vi "Get Alarm Status.vi"(8 "error in (no error)":errorcluster, 9 "Sample Rate Hz":dbl, 10 "Acquisition Metrics in":T1={"Total_Samples"=0, "RPM"=1000.0}, 11 "data":waveform(dbl)[](array[waveform])) -> (0 "error out":errorcluster, 3 "Alarms":T2)   [LabVIEW 2026, in "Acquisition.lvlib"]
uses:
  Acquisition.lvlib
  Controls/Alarms.ctl
  Controls/Frequency Type.ctl
  Controls/Acquisition Metrics.ctl
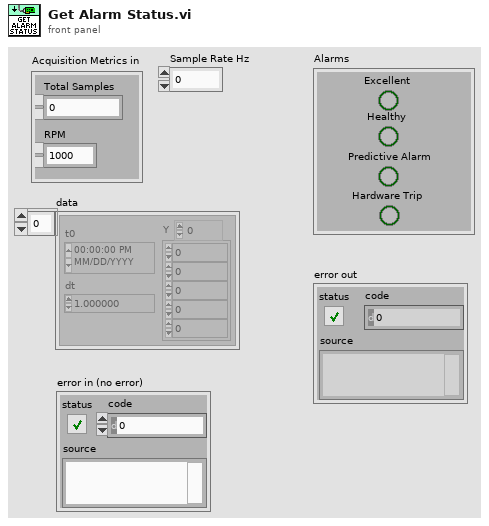
[diagram p1: front panel]
types:
  T1 = typedef "Acquisition.lvlib/Acquisition Metrics.ctl" = cluster{"Total_Samples":i64, "RPM":dbl}
  T2 = typedef "Acquisition.lvlib/Alarms.ctl" = cluster{"Excellent":bool, "Healthy":bool, "Predictive Alarm":bool, "Hardware Trip":bool}
  T3 = typedef "Acquisition.lvlib/Frequency Type.ctl" = enum16{"Calc F_1X", "Calc F_cutoff"}
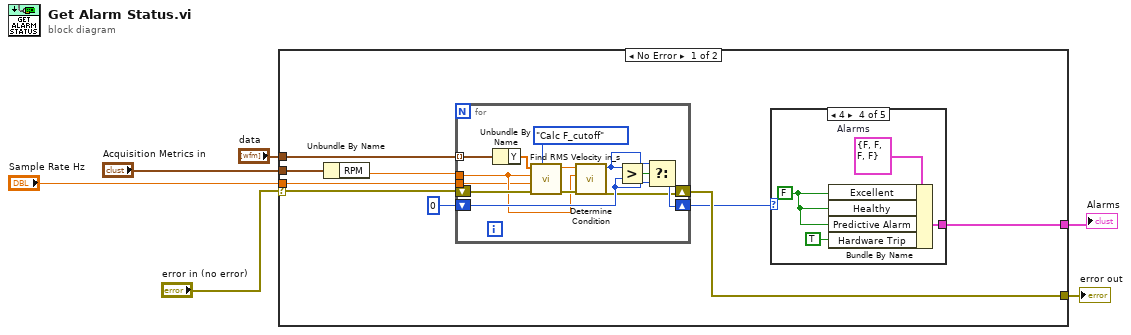
[diagram p0: block diagram]
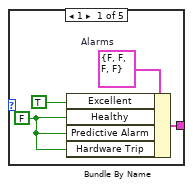
[diagram p2: hidden frame]
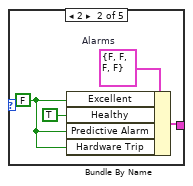
[diagram p3: hidden frame]
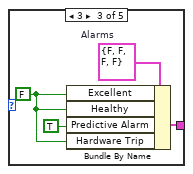
[diagram p4: hidden frame]
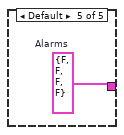
[diagram p5: hidden frame]
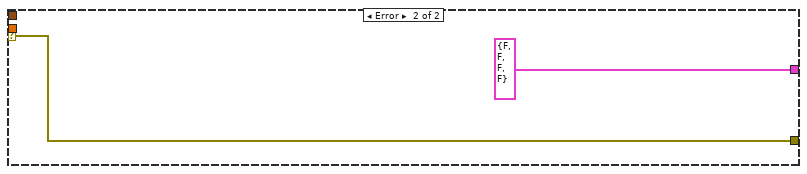
[diagram p6: hidden frame]
diagram:
  n1 = case shown="No Error" "error in (no error)" {
    selector: "error in (no error)" -> [w10 w46]
    tunnel: [w15 w46] -> w6
    tunnel: "data" -> [w14 _]
    tunnel: [w11 T2 {"Excellent"=FALSE, "Healthy"=FALSE, "Predictive Alarm"=FALSE, "Hardware Trip"=FALSE} ("Alarms")] -> w4
    tunnel: "Sample Rate Hz" -> [w9 _]
    tunnel: "Acquisition Metrics in" -> [w8 _]
    frame No Error {
      n2 = Unbundle By Name(w8) -> ("RPM"=w7:dbl)
      n3 = for {
        shift-right: [w24] -> w13
        shift-left: 0 ("Condition") -> [w23]
        tunnel: w14 -> [w21] mode=indexing
        shift-right: [w19] -> w15
        shift-left: w10 -> [w20]
        tunnel: w7 -> [w17]
        tunnel: w9 -> [w16]
        n4 = Unbundle By Name(w21) -> ("Y"=w28:dbl[])
        n5 = call "Find RMS Velocity in_s .vi"("Freq. Type"=Frequency_Type."Calc F_cutoff", "error in (no error)"=w20, "Sample Rate Hz"=w16, "RPM"=w17, "Y"=w28) -> ("error out"=w27:errorcluster, "rms value"=w22:dbl)  [unwired: 5 in]
        n6 = call "Determine Condition.vi"("error in (no error)"=w27, "RPM"=w17, "RMS"=w22) -> ("error out"=w19:errorcluster, "Condition"=w25:i32)  [unwired: 7 in]
        n7 = Greater?(x=w25, y=w23) -> (0:w26:bool)
        n8 = Select(t=w25, s=w26, f=w23) -> (s? t:f=w24:i32)
      }
      n9 = case shown="4" w13 {
        tunnel: [w31 w35 w39 w43 w45] -> w11
        frame 1 {
          w30 = FALSE ("Excellent")
          w32 = T2 {"Excellent"=FALSE, "Healthy"=FALSE, "Predictive Alarm"=FALSE, "Hardware Trip"=FALSE}  # Alarms
          n10 = Bundle By Name(cluster=w32, "Excellent"=TRUE ("Healthy"), "Healthy"=w30, "Predictive Alarm"=w30, "Hardware Trip"=w30) -> (w31:T2)
        }
        frame 2 {
          w34 = FALSE ("Excellent")
          w36 = T2 {"Excellent"=FALSE, "Healthy"=FALSE, "Predictive Alarm"=FALSE, "Hardware Trip"=FALSE}  # Alarms
          n11 = Bundle By Name(cluster=w36, "Excellent"=w34, "Healthy"=TRUE, "Predictive Alarm"=w34, "Hardware Trip"=w34) -> (w35:T2)
        }
        frame 3 {
          w38 = FALSE ("Excellent")
          w40 = T2 {"Excellent"=FALSE, "Healthy"=FALSE, "Predictive Alarm"=FALSE, "Hardware Trip"=FALSE}  # Alarms
          n12 = Bundle By Name(cluster=w40, "Excellent"=w38, "Healthy"=w38, "Predictive Alarm"=TRUE ("Healthy"), "Hardware Trip"=w38) -> (w39:T2)
        }
        frame 4 {
          w41 = FALSE ("Excellent")
          w44 = T2 {"Excellent"=FALSE, "Healthy"=FALSE, "Predictive Alarm"=FALSE, "Hardware Trip"=FALSE}  # Alarms
          n13 = Bundle By Name(cluster=w44, "Excellent"=w41, "Healthy"=w41, "Predictive Alarm"=w41, "Hardware Trip"=TRUE ("Healthy")) -> (w43:T2)
        }
        frame Default {
          w45 = T2 {"Excellent"=FALSE, "Healthy"=FALSE, "Predictive Alarm"=FALSE, "Hardware Trip"=FALSE}  # Alarms
        }
      }
    }
    frame Error {
    }
  }
  "error out" <- w6
  "Alarms" <- w4
